vi "VI Dependent Names.vi"(8 "error in":errorcluster, 10 "SubVI in":refnum<vi>, 11 "Set in":set{string}(c389)) -> (0 "error out":errorcluster, 3 "Set out":set{string}(c389))   [LabVIEW 2020, in "SimpleDependencyInspector.lvlib"]
uses:
  SimpleDependencyInspector.lvlib
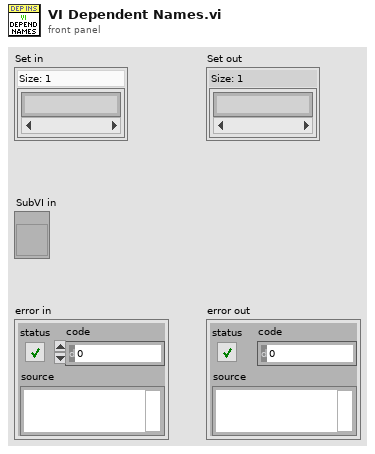
[diagram p1: front panel]
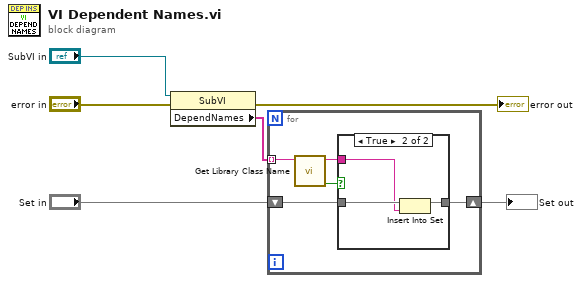
[diagram p0: block diagram]
diagram:
  n1 = property class="SubVI"(reference="SubVI in", error in="error in") -> (error out=→"error out":errorcluster, "DependNames"=w2:string[])  [unwired: 1 out]
  n2 = for {
    tunnel: w2 -> [w11] mode=indexing
    shift-right: [w10] -> w4
    shift-left: "Set in" -> [w9]
    n3 = call "Get Library Class Name.vi"("VI In"=w11) -> ("Found?"=w7:bool, "Name"=w8:string)  [unwired: 9 in]
    n4 = case shown="True" w7 {
      tunnel: [w12 w15] -> w10
      tunnel: w9 -> [w12 w14]
      tunnel: w8 -> [_ w13]
      frame False {
      }
      frame True {
        n5 = Insert Into Set(10:w13, 11:w14) -> (3:w15:set{string})  [unwired: 1 out]
      }
    }
  }
  "Set out" <- w4
